vi "dataflow.vi"() -> ()   [LabVIEW 2018]
panel:
  in  "Numeric 2":dbl
  in  "Numeric":u32
  in  "Temperature (F)":dbl(slide) scale=0.0..200.0
  out "Thermometer (C)":dbl(slide) scale=0.0..100.0
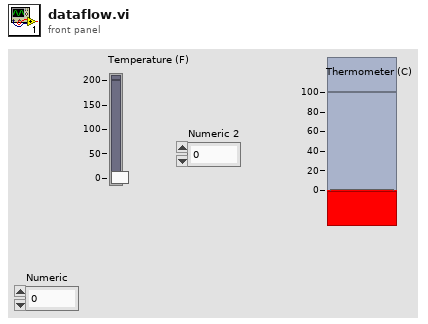
[diagram p1: front panel]
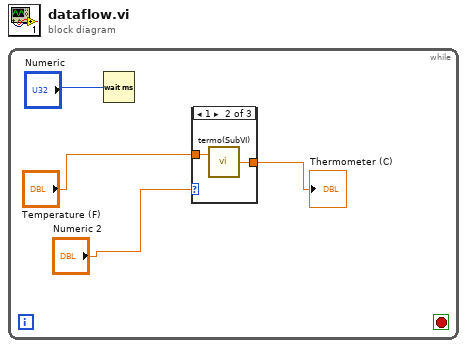
[diagram p0: block diagram]
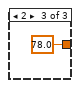
[diagram p3: hidden frame]
diagram:
  n1 = while {
    stop <- w3 stop-if-true
    n2 = Wait (ms)(milliseconds to wait="Numeric") -> ()  [unwired: 1 out]
    n3 = case shown="1" "Numeric 2" {
      tunnel: "Temperature (F)" -> [w6 w8 _]
      tunnel: [w6 w7 78.0 ("Numeric")] -> w4
      frame 0, Default {
      }
      frame 1 {
        n4 = call "termo(SubVI).vi"("Temperature (F)"=w8) -> ("Numeric"=w7:dbl)  [unwired: 1 in]
      }
      frame 2 {
      }
    }
    "Thermometer (C)" <- w4
  }
